vi "edittest save existing sequence.vi"(8 "error in (no error)":errorcluster, 9 "Sequence Fields":T1[](array[typedef]), 10 "Sequence Record In":T4, 11 "Connection Refnum":T5) -> (0 "error out":errorcluster, 2 "Sequence Record":T4, 3 "Connection Refnum":T5)   [LabVIEW 2011]
uses:
  Summitek EXT/ODBC/SQL Controls/Connection Refnum.ctl
  server/database/Sequences/Sequence Record.ctl
  server/database/Fields/Field Record.ctl
  server/database/Fields/Field DataTypes.ctl
  server/database/Fields/Field NextItem.ctl
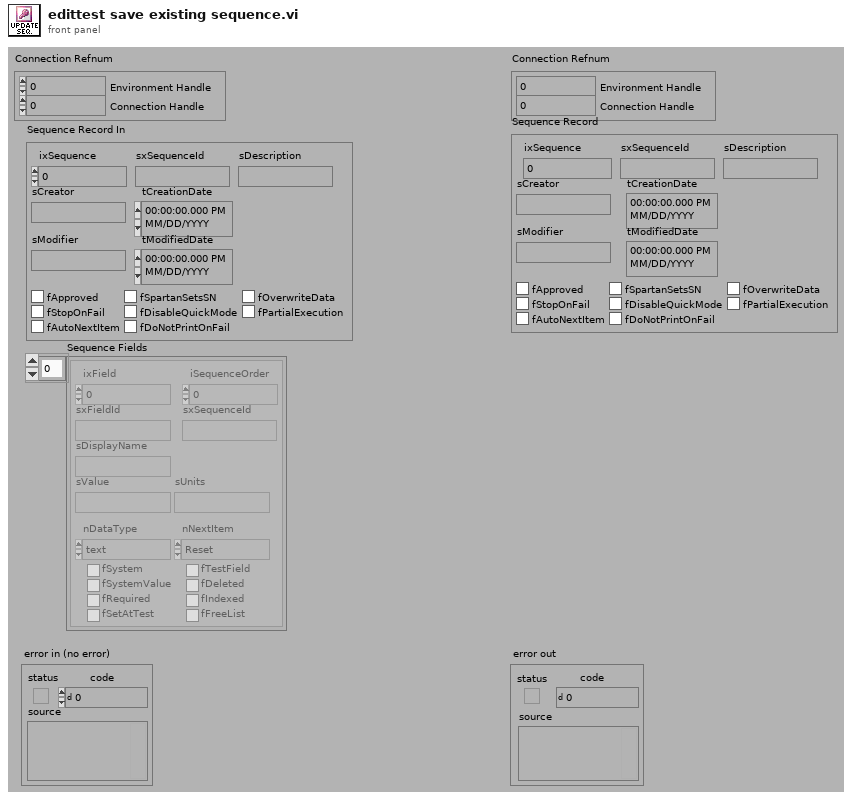
[diagram p1: front panel]
types:
  T1 = typedef "Field Record.ctl" = cluster{"ixField":i32, "iSequenceOrder":i32, "sxFieldId":string, "sxSequenceId":string, "sDisplayName":string, "sValue":string, "sUnits":string, "nDataType":T2, "nNextItem":T3, "fSystem":bool, "fSystemValue":bool, "fRequired":bool, "fSetAtTest":bool, "fTestField":bool, "fDeleted":bool, "fIndexed":bool, "fFreeList":bool}
  T2 = typedef "Field DataTypes.ctl" = enum32{"text", "numeric", "list", "timestamp", "boolean"}
  T3 = typedef "Field NextItem.ctl" = enum32{"Reset", "Retain", "Auto-Increment"}
  T4 = typedef "Sequence Record.ctl" = cluster{"ixSequence":i32, "sxSequenceId":string, "sDescription":string, "sCreator":string, "tCreationDate":timestamp, "sModifier":string, "tModifiedDate":timestamp, "fApproved":bool, "fSpartanSetsSN":bool, "fOverwriteData":bool, "fStopOnFail":bool, "fDisableQuickMode":bool, "fPartialExecution":bool, "fAutoNextItem":bool, "fDoNotPrintOnFail":bool}
  T5 = typedef "Connection Refnum.ctl" = cluster{"Environment Handle":i32, "Connection Handle":i32}
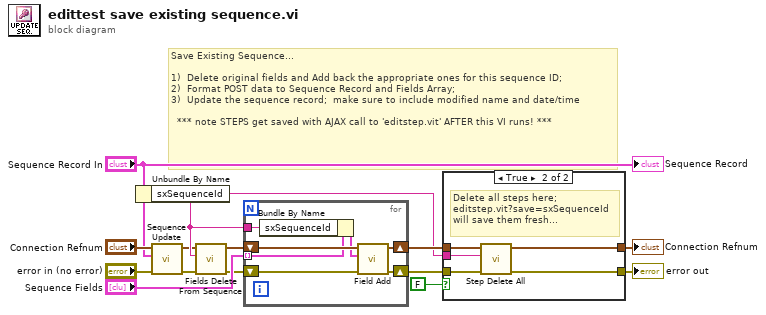
[diagram p0: block diagram]
diagram:
  # "Save Existing Sequence...\n\n1)  Delete original fields and Add back the appropriate ones for this sequence ID;\n2)  Format POST data to Sequence Record and Fields Array;\n3)  Update the sequence record;  make sure to include modified name and date/time\n\n  *** note STEPS get saved with AJAX call to 'editstep.vit' AFTER this VI runs! ***"
  n1 = Unbundle By Name("Sequence Record In") -> ("sxSequenceId"=w9:string)
  n2 = call "Sequence Update.vi"("error in (no error)"="error in (no error)", "Sequence Record"="Sequence Record In", "Connection Refnum"="Connection Refnum") -> ("error out"=w3:errorcluster, "Connection Refnum"=w4:T5)  [unwired: 7 out]
  n3 = call "Fields Delete From Sequence.vi"("error in (no error)"=w3, "sxSequenceId (\"\")"=w9, "Connection Refnum"=w4) -> ("error out"=w12:errorcluster, "Connection Refnum"=w13:T5)  [unwired: 7 out]
  n4 = for {
    shift-right: [w18] -> w11
    shift-left: w13 -> [w21]
    shift-right: [w19] -> w8
    shift-left: w12 -> [w20]
    tunnel: "Sequence Fields" -> [w16] mode=indexing
    tunnel: w9 -> [w17]
    n5 = Bundle By Name(cluster=w16, "sxSequenceId"=w17) -> (w15:T1)
    n6 = call "Field Add.vi"("error in (no error)"=w20, "Field Record"=w15, "Connection Refnum"=w21) -> ("error out"=w19:errorcluster, "Connection Refnum"=w18:T5)  [unwired: 1 in, 6 out]
  }
  n7 = case shown="True" FALSE {
    tunnel: w11 -> [w23 w28]
    tunnel: [w23 w27] -> w10
    tunnel: w9 -> [_ w26]
    tunnel: w8 -> [w22 w25]
    tunnel: [w22 w24] -> w7
    frame False {
    }
    frame True {
      # "Delete all steps here;\neditstep.vit?save=sxSequenceId\nwill save them fresh..."
      n8 = call "Step Delete All.vi"("error in (no error)"=w25, "sxSequenceId (\"\")"=w26, "Connection Refnum"=w28) -> ("error out"=w24:errorcluster, "Connection Refnum"=w27:T5)  [unwired: 7 out]
    }
  }
  "error out" <- w7
  "Connection Refnum" <- w10
  "Sequence Record" <- "Sequence Record In"
